vi "New Actor Data Binding Transport.vi"(7 "Priority (Normal)":T1=enum."Normal", 9 "Datum Return Name":string, 11 "IObserver":refnum<class "Message Enqueuer.lvclass">) -> (0 "error out":errorcluster, 3 "ActorDataBinding out":refnum<class "ActorDataBinding.lvclass">)   [LabVIEW 2017, in "IObserver.lvlib" / "ActorDataBinding.lvclass"]
uses:
  ActorDataBinding.lvclass
  <vilib>/ActorFramework/Message Enqueuer/Message Enqueuer.lvclass
  <vilib>/ActorFramework/Message Enqueuer/Message Priority.ctl
  IObserver Messages/Observe Data Msg/Observe Data Msg.lvclass
  ActorDataBinding.lvclass/ActorDataBinding.ctl
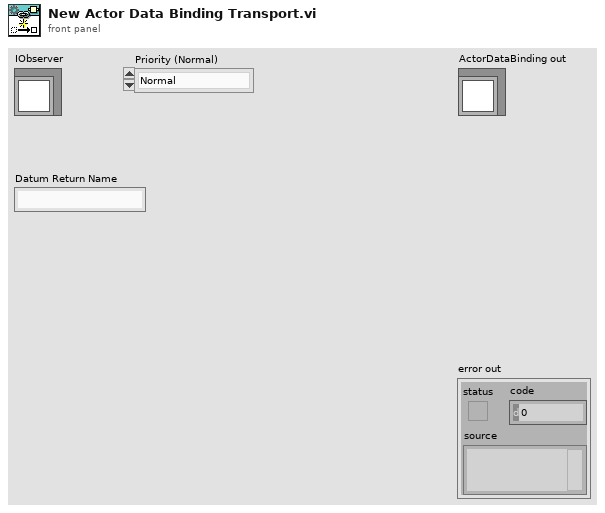
[diagram p1: front panel]
types:
  T1 = typedef "Actor Framework.lvlib/Message Enqueuer.lvclass/Message Priority.ctl" = enum16{"Low", "Normal", "High"}
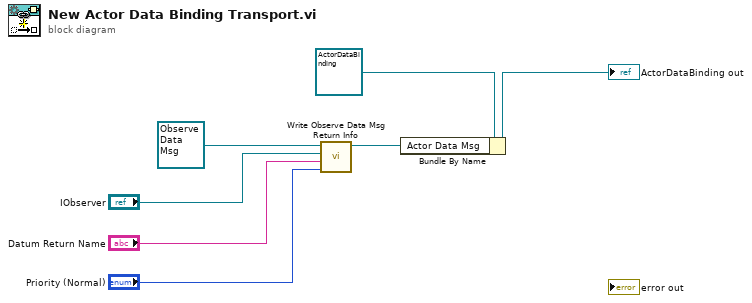
[diagram p0: block diagram]
diagram:
  n1 = call "Write Observe Data Msg Return Info.vi"("Return Priority (Normal)"="Priority (Normal)", "Datum Name"="Datum Return Name", "Message Enqueuer in"="IObserver", "Observe Data Msg In"=refnum<class "Observe Data Msg.lvclass"> refnum ("Transport.lvlib:Actor Data Msg.lvclass")) -> ("Observe Data Msg Out"=w2:refnum<class "Observe Data Msg.lvclass">)  [unwired: 7 in]
  n2 = Bundle By Name(cluster=refnum<class "ActorDataBinding.lvclass"> refnum ("ActorDataBinding in"), "Actor Data Msg"=w2) -> (→"ActorDataBinding out":refnum<class "ActorDataBinding.lvclass">)
